vi "Arguments - Error As Arguments.vi"() -> ()   [LabVIEW 2014]
uses:
  user.lib/_NEVSTOP/Communicable State Machine(CSM)/AdvanceAPI/CSM - Revert Arguments-Safe String.vi
  user.lib/_NEVSTOP/Communicable State Machine(CSM)/_Support/Common/Trim Single line Text.vi
  user.lib/_NEVSTOP/Communicable State Machine(CSM)/AdvanceAPI/CSM - Keywords.vi
  user.lib/_NEVSTOP/Communicable State Machine(CSM)/Communicable State Machine.lvlib
panel:
  out "Arguments":string
  out "error":errorcluster
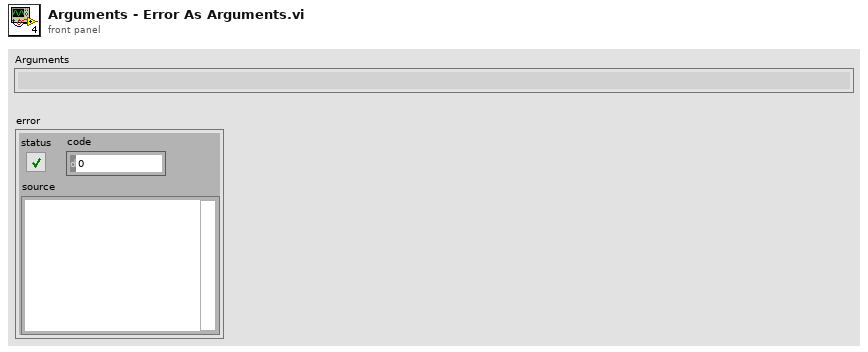
[diagram p1: front panel]
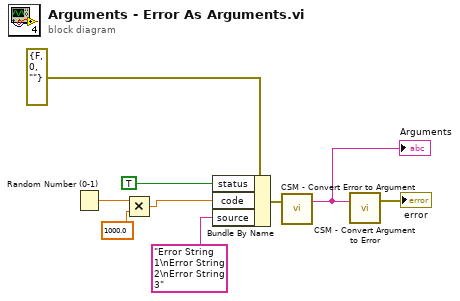
[diagram p0: block diagram]
diagram:
  n1 = Random Number (0-1)() -> (number: 0 to 1=w3:dbl)
  n2 = Multiply(x=w3, y=1000.0) -> (x*y=w2:dbl)
  n3 = Bundle By Name(cluster=errorcluster {"status"=FALSE, "code"=0, "source"=""} ("error constant"), "status"=TRUE, "code"=w2, "source"="Error String 1\nError String 2\nError String 3") -> (w6:errorcluster)
  n4 = call "CSM - Convert Error to Argument.vi"("error in (no error)"=w6) -> ("Arguments"=w5:string)  [unwired: 2 in]
  "Arguments" <- w5
  n5 = call "CSM - Convert Argument to Error.vi"("Argument"=w5) -> ("error"=→"error":errorcluster)  [unwired: 2 in]
